vi "updateScalars.vi"(8 "error in (no error)":errorcluster, 11 "variant":variant) -> (0 "error out":errorcluster)   [LabVIEW 2020, in "ThorlabsWavefrontDS.lvclass"]
uses:
  ThorlabsWavefrontDS.lvclass
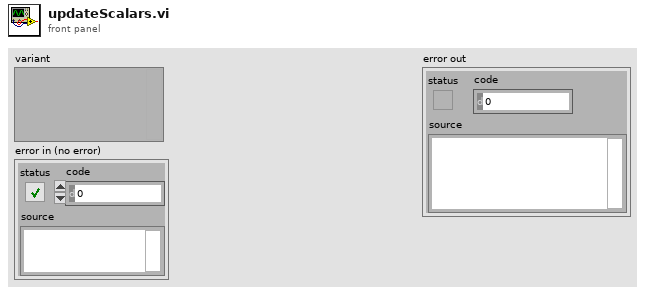
[diagram p1: front panel]
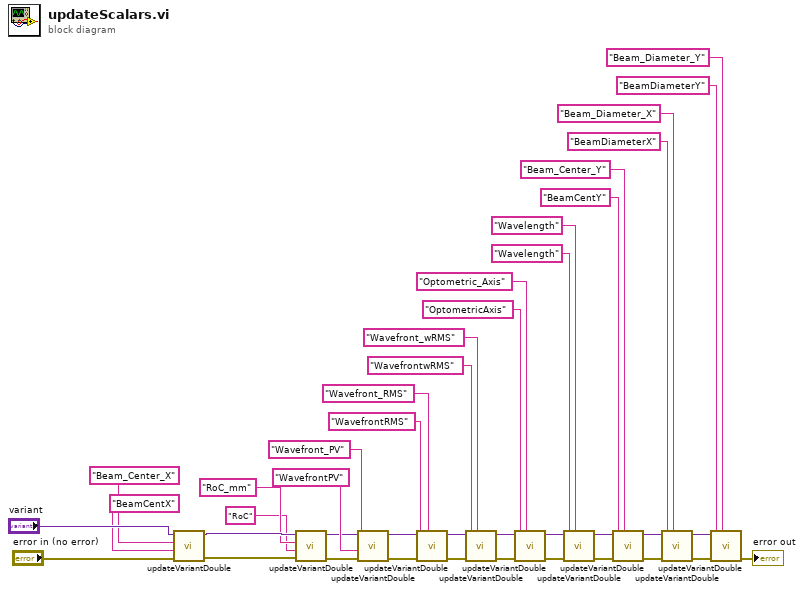
[diagram p0: block diagram]
diagram:
  n1 = call "updateVariantDouble.vi"("error in (no error)"="error in (no error)", "variableName"="BeamCentX", "variantAttrribute"="Beam_Center_X", "variant"="variant") -> ("error out"=w36:errorcluster, "duplicate variant"=w37:variant)  [unwired: 6 in]
  n2 = call "updateVariantDouble.vi"("error in (no error)"=w36, "variableName"="RoC", "variantAttrribute"="RoC_mm", "variant"=w37) -> ("error out"=w31:errorcluster, "duplicate variant"=w30:variant)  [unwired: 6 in]
  n3 = call "updateVariantDouble.vi"("error in (no error)"=w31, "variableName"="WavefrontPV", "variantAttrribute"="Wavefront_PV", "variant"=w30) -> ("error out"=w8:errorcluster, "duplicate variant"=w15:variant)  [unwired: 6 in]
  n4 = call "updateVariantDouble.vi"("error in (no error)"=w8, "variableName"="WavefrontRMS", "variantAttrribute"="Wavefront_RMS", "variant"=w15) -> ("error out"=w7:errorcluster, "duplicate variant"=w14:variant)  [unwired: 6 in]
  n5 = call "updateVariantDouble.vi"("error in (no error)"=w7, "variableName"="WavefrontwRMS", "variantAttrribute"="Wavefront_wRMS", "variant"=w14) -> ("error out"=w6:errorcluster, "duplicate variant"=w13:variant)  [unwired: 6 in]
  n6 = call "updateVariantDouble.vi"("error in (no error)"=w6, "variableName"="OptometricAxis", "variantAttrribute"="Optometric_Axis", "variant"=w13) -> ("error out"=w5:errorcluster, "duplicate variant"=w12:variant)  [unwired: 6 in]
  n7 = call "updateVariantDouble.vi"("error in (no error)"=w5, "variableName"="Wavelength", "variantAttrribute"="Wavelength", "variant"=w12) -> ("error out"=w4:errorcluster, "duplicate variant"=w11:variant)  [unwired: 6 in]
  n8 = call "updateVariantDouble.vi"("error in (no error)"=w4, "variableName"="BeamCentY", "variantAttrribute"="Beam_Center_Y", "variant"=w11) -> ("error out"=w3:errorcluster, "duplicate variant"=w10:variant)  [unwired: 6 in]
  n9 = call "updateVariantDouble.vi"("error in (no error)"=w3, "variableName"="BeamDiameterX", "variantAttrribute"="Beam_Diameter_X", "variant"=w10) -> ("error out"=w2:errorcluster, "duplicate variant"=w9:variant)  [unwired: 6 in]
  n10 = call "updateVariantDouble.vi"("error in (no error)"=w2, "variableName"="BeamDiameterY", "variantAttrribute"="Beam_Diameter_Y", "variant"=w9) -> ("error out"=→"error out":errorcluster)  [unwired: 6 in, 1 out]
